vi "R to T.vi"(11 "Resistance(k)":dbl) -> (3 "Temperature":dbl)   [LabVIEW 2019]
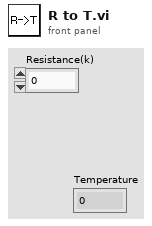
[diagram p1: front panel]
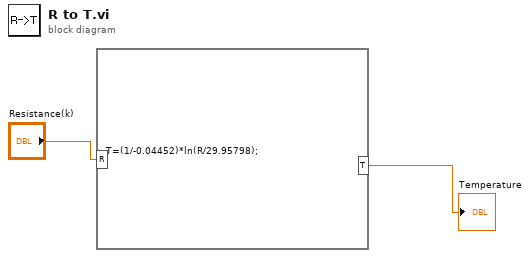
[diagram p0: block diagram]
diagram:
  n1 = formula code="T=(1/-0.04452)*ln(R/29.95798);"("R"="Resistance(k)") -> ("T"=→"Temperature":dbl)
